vi "Random Number Test.vi"() -> ()   [LabVIEW 2025]
panel:
  out "Output Number":u32
  out "Element to change":i32
  out "Player 1 Output":bool[][](array[boolean])
  out "Initialize Array":bool[](array[boolean])
  out "Initial Random Numbers":u8[](array[numeric])
  out "unsigned 8bit integer":u8
  in  "millisecond multiple":u32=100
  in  "Player 1 Input":bool[][](array[boolean])
  out "output array":bool[](array[boolean])
  in  "stop":bool
  out "floor(x): largest int <= x":dbl
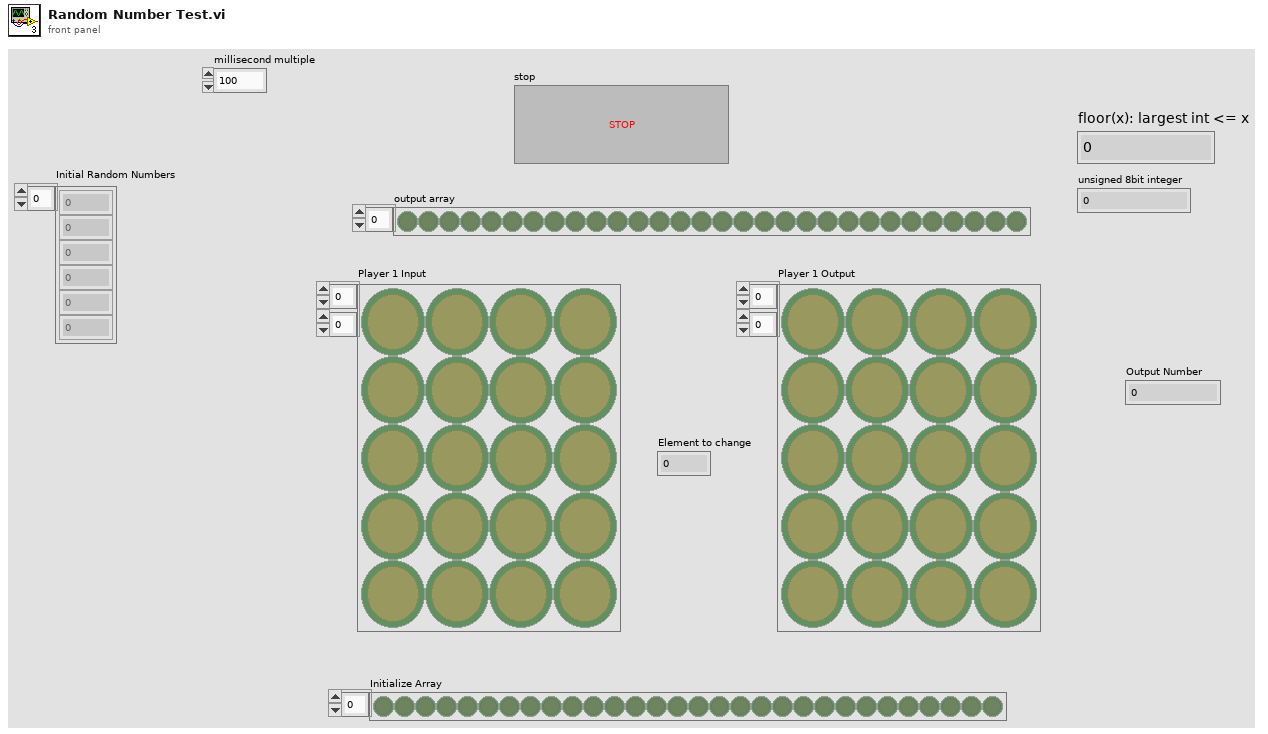
[diagram p1: front panel]
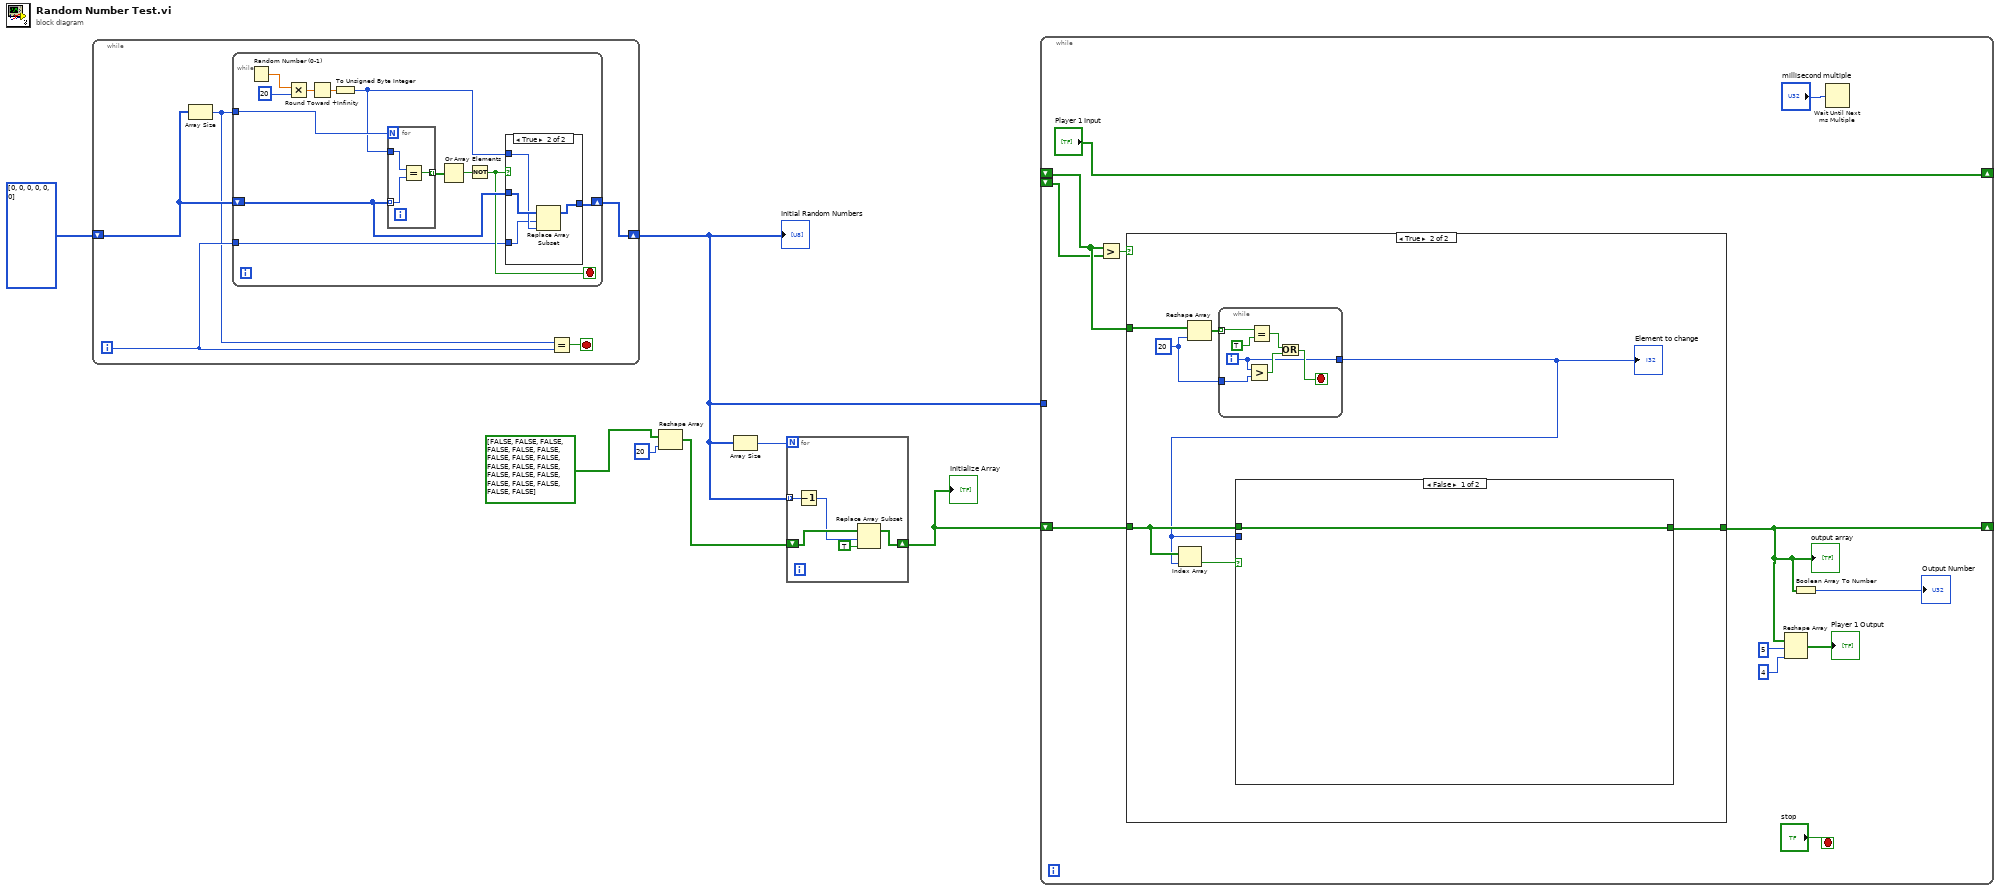
[diagram p0: block diagram]
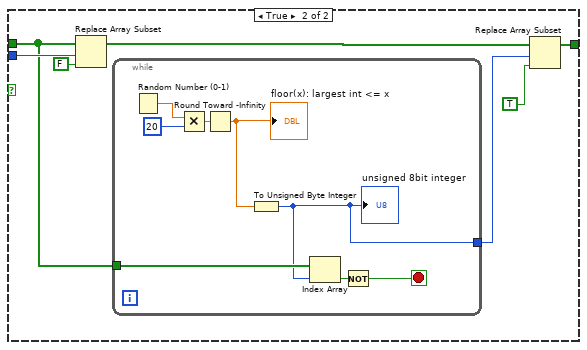
[diagram p4: hidden frame]
diagram:
  n1 = while {
    shift-right: [w8] -> w7
    shift-left: u8[] [0, 0, 0, 0, 0, 0] ("Initial Random Numbers") -> [w10]
    i -> [w12]
    stop <- w11 stop-if-true
    n2 = Array Size(array=w10) -> (size(s)=w9:i32)
    n3 = while {
      tunnel: w12 -> [w13]
      shift-right: [w15] -> w8
      shift-left: w10 -> [w17]
      tunnel: w9 -> [w20]
      stop <- w16 stop-if-true
      n4 = Random Number (0-1)() -> (number: 0 to 1=w22:dbl)
      n5 = Multiply(x=w22, y=i8 20) -> (x*y=w23:dbl)
      n6 = Round Toward +Infinity(x=w23) -> (ceil(x): smallest int >= x=w24:dbl)
      n7 = To Unsigned Byte Integer(number=w24) -> (unsigned 8bit integer=w14:u8)
      n8 = for {
        N: w20 -> [_]
        tunnel: w17 -> [w31] mode=indexing
        tunnel: w14 -> [w32]
        tunnel: [w30] -> w19 mode=indexing
        n9 = Equal?(x=w32, y=w31) -> (x = y?=w30:bool)
      }
      n10 = Or Array Elements(Boolean array=w19) -> (logical OR=w18:bool)
      n11 = Not(x=w18) -> (.not. x?=w16:bool)
      n12 = case shown="True" w16 {
        tunnel: w17 -> [w25 w29]
        tunnel: [w25 w28] -> w15
        tunnel: w14 -> [_ w27]
        tunnel: w13 -> [_ w26]
        frame False {
        }
        frame True {
          n13 = Replace Array Subset(array=w29, new element=w27, index=w26) -> (w28:u8[])
        }
      }
    }
    n14 = Equal?(x=w9, y=w12) -> (x = y?=w11:bool)
  }
  "Initial Random Numbers" <- w7
  n15 = Reshape Array(bool[][] [[FALSE, FALSE, FALSE, FALSE], [FALSE, FALSE, FALSE, FALSE], [FALSE, FALSE, FALSE, FALSE], [FALSE, FALSE, FALSE, FALSE], [FALSE, FALSE, FALSE, FALSE]] ("Player 1"), 20 ("dimension size")) -> (w3:bool[])
  n16 = Array Size(array=w7) -> (size(s)=w6:i32)
  n17 = for {
    N: w6 -> [_]
    tunnel: w7 -> [w34] mode=indexing
    shift-right: [w37] -> w2
    shift-left: w3 -> [w36]
    n18 = Decrement(x=w34) -> (x-1=w33:u8)
    n19 = Replace Array Subset(array=w36, new element=TRUE ("new element/subarray"), index=w33) -> (w37:bool[])
  }
  "Initialize Array" <- w2
  n20 = while {
    shift-right: [w41] -> _
    shift-left: w2 -> [w44]
    shift-right: ["Player 1 Input"] -> _
    shift-left: _ -> [w39]
    tunnel: w7 -> [_]
    shift-left: _ -> [w38]
    stop <- "stop" stop-if-true
    n21 = Greater?(x=w39, y=w38) -> (0:w43:bool)
    n22 = case shown="True" w43 {
      tunnel: [w50 w54] -> w41
      tunnel: w44 -> [w50 w53]
      tunnel: w39 -> [_ w57]
      frame False {
      }
      frame True {
        w55 = 20 ("dimension size")
        n23 = Reshape Array(w57, w55) -> (w56:bool[])
        n24 = while {
          tunnel: w56 -> [w80] mode=indexing
          tunnel: w55 -> [w76]
          tunnel: [w74] -> w52
          i -> [w74]
          stop <- w77 stop-if-true
          n25 = Greater?(x=w74, y=w76) -> (0:w75:bool)
          n26 = Equal?(x=w80, y=TRUE ("element")) -> (x = y?=w78:bool)
          n27 = Or(x=w78, y=w75) -> (x .or. y?=w77:bool)
        }
        "Element to change" <- w52
        n28 = Index Array(array=w53, index=w52) -> (element=w51:bool)
        n29 = case shown="False" w51 {
          tunnel: w52 -> [_ w65]
          tunnel: [w58 w61] -> w54
          tunnel: w53 -> [w58 w59]
          frame False {
          }
          frame True {
            n30 = Replace Array Subset(array=w59, new element=FALSE ("new element/subarray"), index=w65) -> (w63:bool[])
            n31 = while {
              tunnel: [w66] -> w60
              tunnel: w59 -> [w69]
              stop <- w67 stop-if-true
              n32 = Random Number (0-1)() -> (number: 0 to 1=w72:dbl)
              n33 = Multiply(x=w72, y=i8 20) -> (x*y=w73:dbl)
              n34 = Round Toward -Infinity(1:w73) -> (0:w70:dbl)
              "floor(x): largest int <= x" <- w70
              n35 = To Unsigned Byte Integer(number=w70) -> (unsigned 8bit integer=w66:u8)
              "unsigned 8bit integer" <- w66
              n36 = Index Array(array=w69, index=w66) -> (element=w68:bool)
              n37 = Not(x=w68) -> (.not. x?=w67:bool)
            }
            n38 = Replace Array Subset(array=w63, new element=TRUE ("new element/subarray"), index=w60) -> (w61:bool[])
          }
        }
      }
    }
    "output array" <- w41
    n39 = Reshape Array(w41, 5 ("dimension size"), 4 ("dimension size")) -> (→"Player 1 Output":bool[][])
    n40 = Boolean Array To Number(Boolean array=w41) -> (number=→"Output Number":u32)
    n41 = Wait Until Next ms Multiple(millisecond multiple="millisecond multiple") -> ()  [unwired: 1 out]
  }
